vi "读取定时器.vi"(8 "error in (no error)":errorcluster caption="错误输入（无错误）", 11 "定时器类 输入":refnum<class "定时器类.lvclass">) -> (0 "error out":errorcluster caption="错误输出", 1 "定时到脉冲":bool, 2 "定时到":bool, 3 "定时器类 输出":refnum<class "定时器类.lvclass">, 4 "经历时间":u32)   [LabVIEW 2014, in "定时器类.lvclass"]
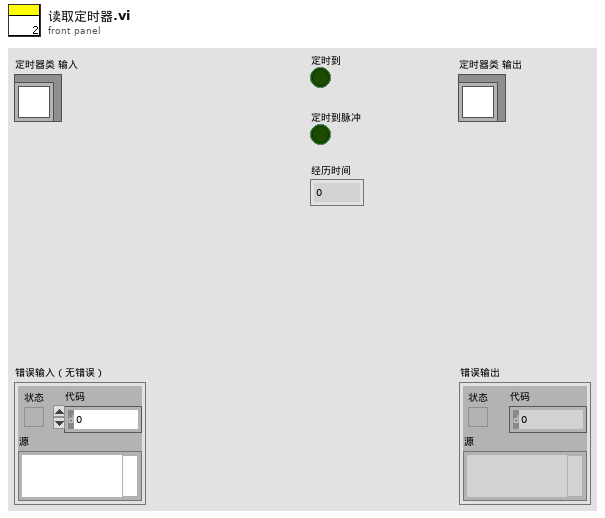
[diagram p1: front panel]
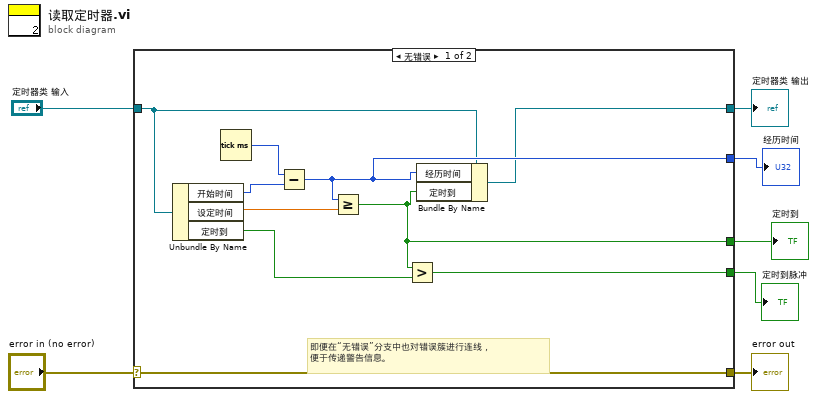
[diagram p0: block diagram]
diagram:
  n1 = case shown="无错误" "error in (no error)" {
    selector: "error in (no error)" -> [w17 w19]
    tunnel: [w17 w19] -> w6
    tunnel: [w8 w18] -> w4
    tunnel: "定时器类 输入" -> [w9 w18]
    tunnel: [w12 _] -> w3
    tunnel: [w11 _] -> w2
    tunnel: [w10 _] -> w1
    frame No Error {
      # "即便在“无错误”分支中也对错误簇进行连线，\n便于传递警告信息。"
      n2 = Unbundle By Name(w9) -> ("开始时间"=w15:u32, "设定时间"=w14:dbl, "定时到"=w13:bool)
      n3 = Tick Count (ms)() -> (millisecond timer value=w16:u32)
      n4 = Subtract(x=w16, y=w15) -> (x-y=w10:u32)
      n5 = Greater Or Equal?(x=w10, y=w14) -> (x >= y?=w12:bool)
      n6 = Greater?(x=w12, y=w13) -> (0:w11:bool)
      n7 = Bundle By Name(cluster=w9, "经历时间"=w10, "定时到"=w12) -> (w8:refnum<class "定时器类.lvclass">)
    }
    frame Error {
    }
  }
  "error out" <- w6
  "定时器类 输出" <- w4
  "定时到" <- w3
  "定时到脉冲" <- w2
  "经历时间" <- w1
